vi "AE Variables_bak.vi"(6 "AcqFilt":T1, 7 "Action":T2=enum."Set Blue Pressure", 8 "error in (no error)":errorcluster, 9 "Height In":dbl, 10 "Pressure In":dbl, 11 "Filter In":bool=TRUE) -> (0 "error out":errorcluster, 1 "Height Out":dbl, 2 "Pressure Out":dbl, 3 "Filter Out":bool=TRUE, 4 "AcqFilt 2":T1 caption="AcqFilt")   [LabVIEW 2013]
uses:
  Controls/Enum Variables.ctl
  Controls/Enum AcqFilter.ctl
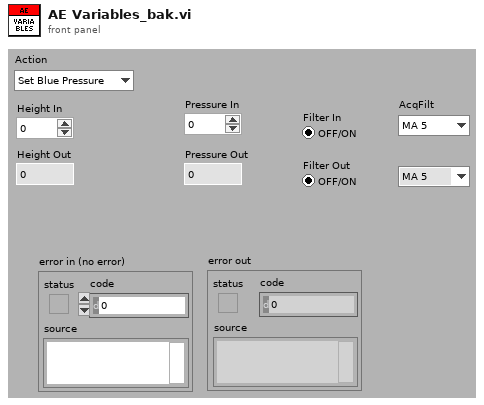
[diagram p1: front panel]
types:
  T1 = typedef "Medimatic.lvlib/Enum AcqFilter.ctl" = enum16{"MA 5", "MA 8", "Hanning"}
  T2 = typedef "Medimatic.lvlib/Enum Variables.ctl" = enum16{"SetAcqFilter", "GetAcqFilter", "Set Filter", "Get Filter", "Set Height", "Get Height", "Set Blue Pressure", "Get Blue Pressure", "Set Red Pressure", "Get Red Pressure", "Init", "Reset Pressure"}
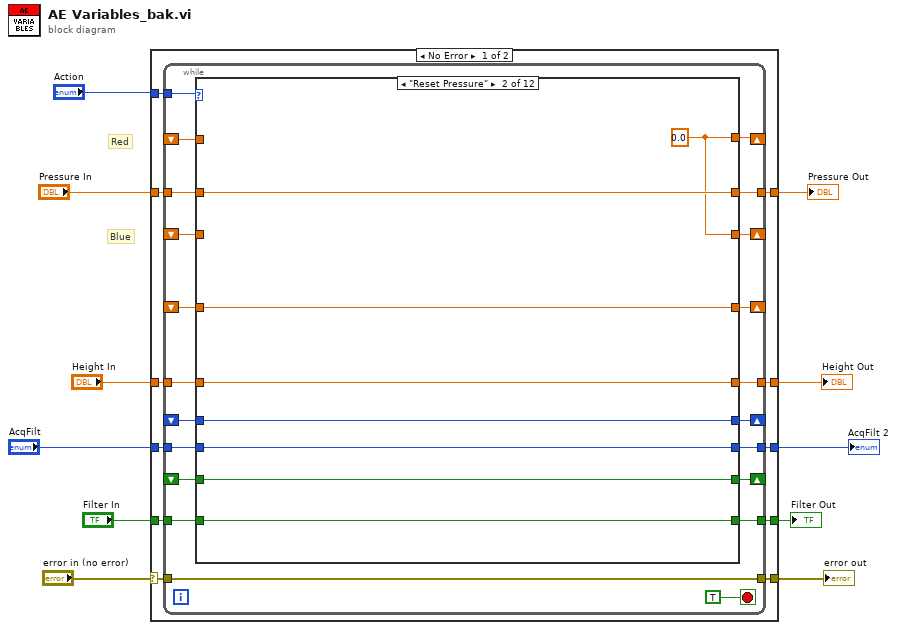
[diagram p0: block diagram]
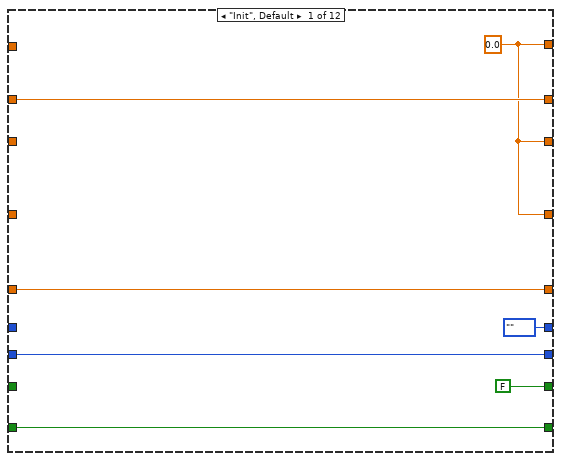
[diagram p2: hidden frame]
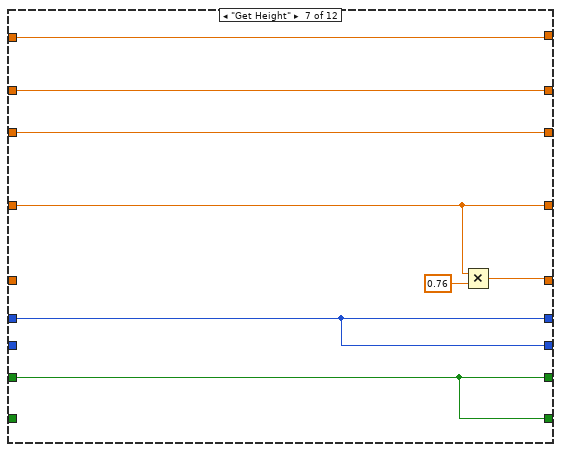
[diagram p7: hidden frame]
diagram:
  # "Blue"
  # "Red"
  n1 = case shown="No Error" "error in (no error)" {
    selector: "error in (no error)" -> [w19 w141]
    tunnel: "Action" -> [w22 _]
    tunnel: "Pressure In" -> [w21 w140]
    tunnel: [w20 w140] -> w10
    tunnel: [w18 w141] -> w8
    tunnel: "Height In" -> [w17 w139]
    tunnel: [w16 w139] -> w5
    tunnel: "Filter In" -> [w15 w138]
    tunnel: [w14 w138] -> w3
    tunnel: "AcqFilt" -> [w13 w137]
    tunnel: [w12 w137] -> w1
    frame No Error {
      n2 = while {
        shift-right: [w41] -> _
        shift-left: _ -> [w42]
        tunnel: w22 -> [w43]
        tunnel: w21 -> [w40]
        tunnel: [w39] -> w20
        tunnel: w19 -> [w38]
        tunnel: [w38] -> w18
        shift-right: [w36] -> _
        shift-left: _ -> [w35]
        shift-right: [w33] -> _
        shift-left: _ -> [w32]
        tunnel: w17 -> [w34]
        tunnel: [w31] -> w16
        shift-right: [w29] -> _
        shift-left: _ -> [w30]
        tunnel: w15 -> [w28]
        tunnel: [w27] -> w14
        tunnel: w13 -> [w26]
        tunnel: [w25] -> w12
        shift-right: [w24] -> _
        shift-left: _ -> [w23]
        stop <- TRUE stop-if-true
        n3 = case shown="\"Reset Pressure\"" w43 {
          tunnel: [w49 w57 w66 w74 w81 w90 w98 w106 w114 w121 w129 w136] -> w41
          tunnel: w42 -> [_ _ _ w74 w81 w90 w98 w106 w114 w121 w129 w136]
          tunnel: w40 -> [w50 w58 w66 _ w82 _ w97 w105 w113 w120 w128 w135]
          tunnel: [w50 w58 w66 w74 w82 w89 w97 w105 w113 w120 w128 w135] -> w39
          tunnel: [w49 w57 w65 w73 w82 w89 w96 w104 w112 w119 w127 w134] -> w36
          tunnel: w35 -> [_ _ w65 w73 _ w89 w96 w104 w112 w119 w127 w134]
          tunnel: w34 -> [w48 w56 w63 w71 w79 w87 _ w103 w111 w118 w126 w133]
          tunnel: [w49 w55 w64 w72 w80 w88 w93 w103 w110 w116 w124 w131] -> w33
          tunnel: w32 -> [_ w55 w64 w72 w80 w88 w93 _ w110 w116 w124 w131]
          tunnel: [w48 w56 w63 w71 w79 w87 w94 w103 w111 w118 w126 w133] -> w31
          tunnel: w30 -> [_ w54 w62 w70 w78 w86 w95 w102 w109 _ w123 _]
          tunnel: [FALSE ("Filter In") w54 w62 w70 w78 w86 w95 w102 w109 w117 w123 w132] -> w29
          tunnel: w28 -> [w47 w53 w61 w69 w77 w85 _ w101 _ w117 w125 w132]
          tunnel: [w47 w53 w61 w69 w77 w85 w95 w101 w109 w117 w125 w132] -> w27
          tunnel: w26 -> [w45 w52 w60 w68 w76 w84 _ w100 w108 w115 _ w130]
          tunnel: [w45 w52 w60 w68 w76 w84 w91 w100 w108 w115 w122 w130] -> w25
          tunnel: [enum16{""}."" ("AcqFiltIn") w51 w59 w67 w75 w83 w91 w99 w107 w115 w122 w130] -> w24
          tunnel: w23 -> [_ w51 w59 w67 w75 w83 w91 w99 w107 _ w122 _]
          frame "Init", Default {
            w49 = 0.0 ("Event In")
          }
          frame "Reset Pressure" {
            w57 = 0.0 ("Event In")
          }
          frame "Set Red Pressure" {
          }
          frame "Get Red Pressure" {
          }
          frame "Set Blue Pressure" {
          }
          frame "Get Blue Pressure" {
          }
          frame "Get Height" {
            n4 = Multiply(x=w93, y=0.76) -> (x*y=w94:dbl)
          }
          frame "Set Height" {
          }
          frame "Get Filter" {
          }
          frame "Set Filter" {
          }
          frame "GetAcqFilter" {
          }
          frame "SetAcqFilter" {
          }
        }
      }
    }
    frame Error {
    }
  }
  "Pressure Out" <- w10
  "error out" <- w8
  "Height Out" <- w5
  "Filter Out" <- w3
  "AcqFilt 2" <- w1
